vi "CONST_DST.vi"() -> (2 "DST":i32)   [LabVIEW 2018]
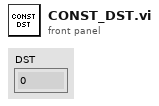
[diagram p1: front panel]
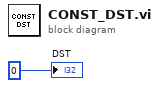
[diagram p0: block diagram]
diagram:
  "DST" <- 0 ("DST")
